vi "Loss-of-Comm Monitor.vi"(8 "Error In":errorcluster, 9 "Host to Ping":string, 11 "CTO!":refnum<notifier>) -> (0 "Error Out":errorcluster, 3 "CTO! Out":refnum<notifier>)   [LabVIEW 2018]
uses:
  Ping Reply Info.ctl
  Instance          10 28Saved   Loss-of-Comm Monitor .vi
  Instance           7 28Saved   Loss-of-Comm Monitor .vi
panel:
  in  "Tab":enum32{"Status", "Details"}(tab)
  out "CTO DownTime":dbl caption="Connection\nDown Time" format="%<%H:%M:%S>t"
  out "CTO Now?":bool caption="Connection:"
  out "PTO Current":bool caption="Current Status:\nLast Ping:"
  in  "Clear":bool
  out "CTO Time":timestamp caption="Connection Lost At:" format="%<%.1X\n%x>T"
  out "PTO Time":timestamp caption="Last Ping Lost At:" format="%<%.1X\n%x>T"
  out "CTO Latched?":bool caption="Connection \nTimed Out?"
  out "PTO Latched?":bool caption="Latched Status:\nPing Timed Out?"
  in  "Connection \nTimeout":u32=1000
  in  "Ping Timeout":i32=300
  in  "Restart":bool
  in  "Stop":bool
  out "Status":string
  out "Chart":i32(graph) caption="Ping Target: [10.6.6.1]"
  out "Last Error Out":errorcluster
  in  "ReTxDelay":u32=200
  out "RxCount":i32 caption="Packets Received"
  out "RxBytes":i32 caption="Bytes\nReceived\nBack"
  in  "Sequence Number":u16 format="%04x"
  out "Ping Reply Info":T1 {"Sequence" format="%04x"}
  out "Socket Out":u32 caption="Socket ID Obtained" format="%04x"
  out "Resolved Host IP":u32 format="%x"
  out "Bytes Sent":i32
  in  "Data Size in Bytes (32)":i32=8
  in  "TTL":u8=128 min=1
  out "LVT":u32
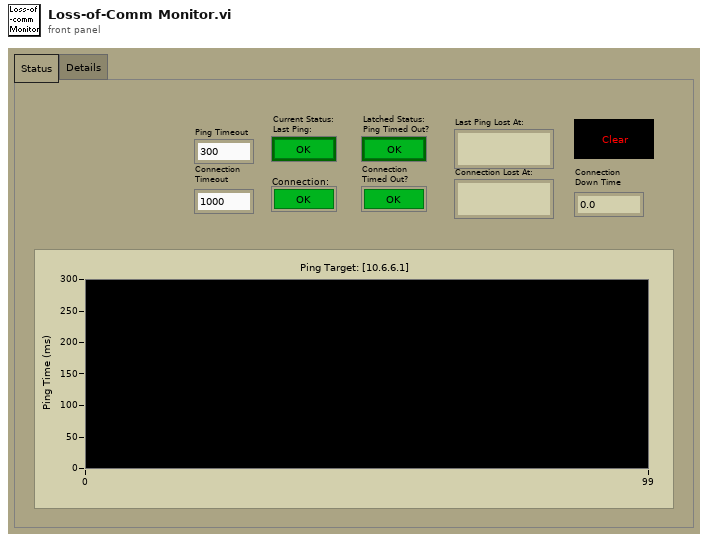
[diagram p1: front panel]
types:
  T1 = typedef "Ping Reply Info.ctl" = cluster{"Source Address":string, "Bytes":i32, "Sequence":u16, "Time (ms)":i32, "Hops":u8, "TTL Returned":u8, "Status":string}
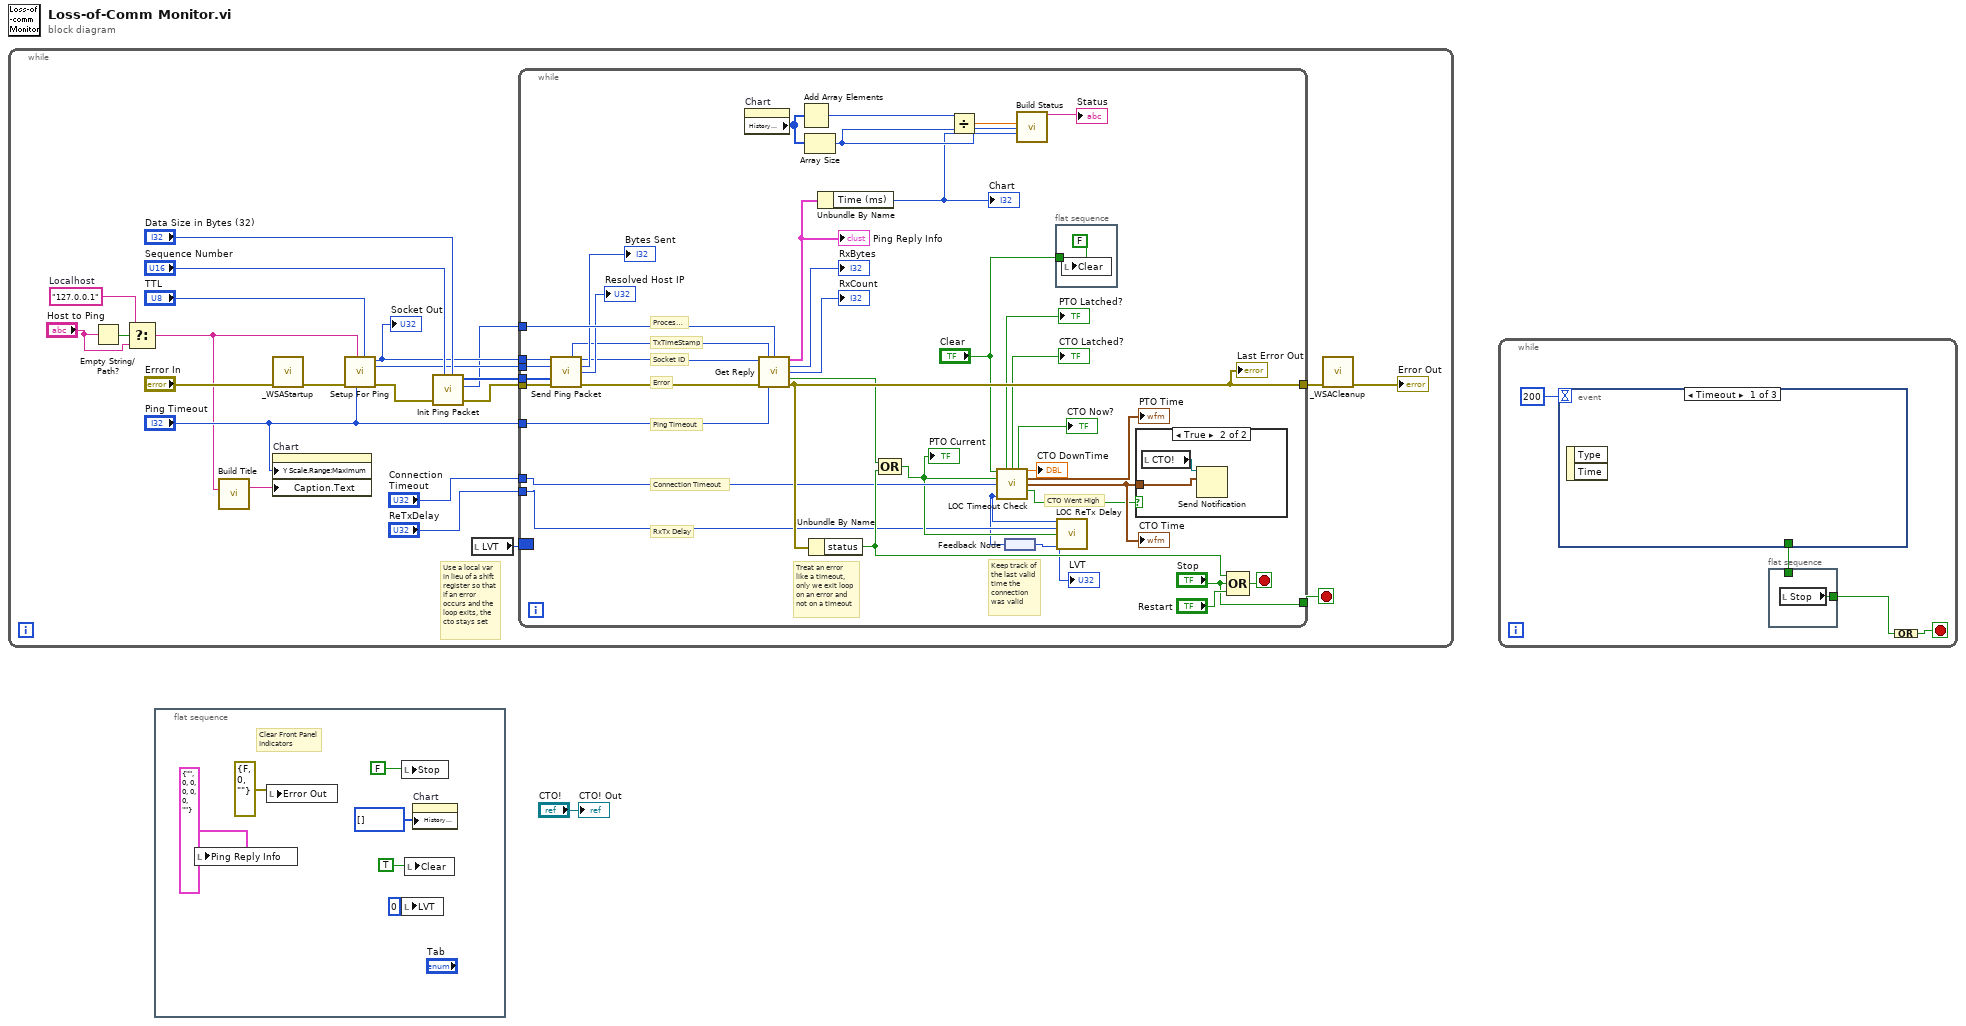
[diagram p0: block diagram]
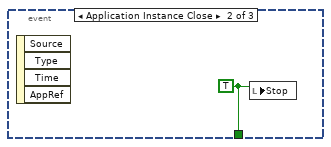
[diagram p2: hidden frame]
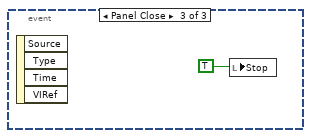
[diagram p3: hidden frame]
diagram:
  n1 = while {
    stop <- w11 stop-if-true
    w3 = "127.0.0.1"  # Localhost
    # "Use a local var\nin lieu of a shift\nregister so that\nif an error\noccurs and the\nloop exits, the\ncto stays set"
    n2 = Empty String/Path?(string/path="Host to Ping") -> (empty?=w5:bool)
    n3 = Select(t=w3, s=w5, f="Host to Ping") -> (s? t:f=w2:string)
    n4 = call "Build Title"("Host"=w2) -> ("Result"=w6:string)  [unwired: 13 in, 1 out]
    n5 = call "_WSAStartup.vi"("Error In"="Error In") -> ("Error out"=w24:errorcluster)  [unwired: 9 in, 1 out]
    n6 = property on="Chart" class="WFChart (strict)"("Y Scale.Range:Maximum"="Ping Timeout", "Caption.Text"=w6) -> ()  [unwired: 2 in, 2 out]
    n7 = call "Setup For Ping.vi"("TTL (U8)"="TTL", "Timeout (ms)"="Ping Timeout", "Host to Ping"=w2, "Error In"=w24) -> ("Error Out"=w23:errorcluster, "Resolved IP"=w16:u32, "Socket Out"=w15:u32)  [unwired: 5 in]
    "Socket Out" <- w15
    n8 = call "Init Ping Packet.vi"("Data Size in Bytes (32)"="Data Size in Bytes (32)", "Sequence Number"="Sequence Number", "Error In"=w23) -> ("Error Out"=w22:errorcluster, "ProcessID"=w13:u32, "Output Packet"=w14:u8[])  [unwired: 6 in]
    n9 = local read "LVT"() -> (w7:u32)
    n10 = while {
      tunnel: w22 -> [w63]
      tunnel: w16 -> [w62]
      tunnel: w15 -> [w61]
      tunnel: w14 -> [w60]
      tunnel: "Ping Timeout" -> [w59]
      tunnel: w13 -> [w58]
      tunnel: [w39] -> w12
      tunnel: ["Stop"] -> w11
      tunnel: "ReTxDelay" -> [w30]
      tunnel: "Connection \nTimeout" -> [w37]
      border: w7 -> [_]
      stop <- w49 stop-if-true
      # "CTO Went High"
      # "Keep track of\nthe last valid\ntime the\nconnection\nwas valid"
      # "RxTx Delay"
      # "Connection Timeout"
      # "Treat an error \nlike a timeout,\nonly we exit loop\non an error and\nnot on a timeout"
      # "Error"
      # "Ping Timeout"
      # "TxTimeStamp"
      # "Socket ID"
      # "ProcessID"
      n11 = call "Send Ping Packet.vi"("Socket To Use"=w61, "Resolved Host IP"=w62, "Packet to Send"=w60, "Error In"=w63) -> ("TxTimeStamp"=w51:u32, "Socket To Use Out"=w53:u32, "Bytes Sent"=→"Bytes Sent":i32, "Resolved Host IP Out"=→"Resolved Host IP":u32, "Error Out"=w52:errorcluster)  [unwired: 7 in]
      n12 = property on="Chart" class="WFChart (strict)"() -> ("History Data"=w47:i32[])  [unwired: 2 in, 2 out]
      n13 = call "Get Reply.vi"("Socket"=w53, "TxTimeStamp Alt"=w51, "ProcessID"=w58, "Error In"=w52, "Timeout (ms)"=w59) -> ("Ping Reply Info"=w50:T1, "RxBytes"=→"RxBytes":i32, "RxCount"=→"RxCount":i32, "Timed Out?"=w32:bool, "Error Out"=w39:errorcluster)  [unwired: 6 in]
      "Ping Reply Info" <- w50
      "Last Error Out" <- w39
      n14 = Add Array Elements(numeric array=w47) -> (sum=w48:i32)
      n15 = Array Size(array=w47) -> (size(s)=w44:i32)
      n16 = Unbundle By Name(w39) -> ("status"=w40:bool)
      n17 = Unbundle By Name(w50) -> ("Time (ms)"=w38:i32)
      "Chart" <- w38
      n18 = Compound Arithmetic op=OR(w32, w40) -> (w31:bool)
      "PTO Current" <- w31
      n19 = Divide(x=w48, y=w44) -> (x/y=w46:dbl)
      n20 = feedback #1() -> (w28:u32)
      n21 = call "LOC Timeout Check.vi"("Clear?"="Clear", "Ping Time Out?"=w31, "Connection Timeout"=w37, "Last Valid TimeStamp"=w28) -> ("PTO Latched"=→"PTO Latched?":bool, "CTO Latched"=→"CTO Latched?":bool, "CTO Current"=→"CTO Now?":bool, "CTO Total Time"=→"CTO DownTime":dbl, "Last PTO Time"=→"PTO Time":timestamp, "CTO Start Time"=w33:timestamp, "CTO Positive Edge"=w26:bool)  [unwired: 5 in]
      "CTO Time" <- w33
      n22 = call "Build Status"("Avg"=w46, "#"=w44, "Current"=w38) -> ("Result"=→"Status":string)  [unwired: 11 in, 1 out]
      n23 = flat-sequence {
        tunnel: "Clear" -> [_]
        frame #0 {
          n24 = local write "Clear"(FALSE ("Clear")) -> ()
        }
      }
      n25 = call "LOC ReTx Delay.vi"("Last Valid In"=w28, "ReTxDelay"=w30, "Ping Time Out?"=w31) -> ("Last Valid Out"=w27:u32)  [unwired: 12 in]
      "LVT" <- w27
      n26 = feedback-in #1(w27) -> ()
      n27 = case shown="True" w26 {
        tunnel: w33 -> [_ w65]
        frame False {
        }
        frame True {
          n28 = local read "CTO!"() -> (w64:refnum<notifier>)
          n29 = Send Notification(notification=w65, notifier=w64) -> ()  [unwired: 1 in, 2 out]
        }
      }
      n30 = Compound Arithmetic op=OR(w40, "Stop", "Restart") -> (w49:bool)
    }
    n31 = call "_WSACleanup.vi"("Error In"=w12) -> ("Error Out"=→"Error Out":errorcluster)  [unwired: 10 in]
  }
  n32 = flat-sequence {
    frame #0 {
      # "Clear Front Panel\nIndicators"
      n33 = local write "Ping Reply Info"(T1 {"Source Address"="", "Bytes"=0, "Sequence"=0, "Time (ms)"=0, "Hops"=0, "TTL Returned"=0, "Status"=""} ("Ping Reply Info")) -> ()
      n34 = local write "Error Out"(errorcluster {"status"=FALSE, "code"=0, "source"=""} ("Error Out")) -> ()
      n35 = local write "Stop"(FALSE ("End")) -> ()
      n36 = local write "LVT"(u32 0 ("LVT")) -> ()
      n37 = local write "Clear"(TRUE ("Clear")) -> ()
      n38 = property on="Chart" class="WFChart (strict)"("History Data"=i32[] []) -> ()  [unwired: 2 in, 2 out]
    }
  }
  n39 = while {
    stop <- w76 stop-if-true
    n40 = event shown="[0] Timeout" {
      selector: _ -> [_ _ _]
      dyn-events: _ -> [_ _ _]
      timeout: 200 -> [_ _ _]
      tunnel: [_ w78 _] -> w73
      event Timeout {
        n41 = event-data() -> ()  [unwired: 1 in, 2 out]
      }
      event Application Instance Close {
        w78 = TRUE ("End")
        n42 = event-data() -> ()  [unwired: 1 in, 4 out]
        n43 = local write "Stop"(w78) -> ()
      }
      event Panel Close {
        n44 = event-data() -> ()  [unwired: 1 in, 4 out]
        n45 = local write "Stop"(TRUE ("End")) -> ()
      }
    }
    n46 = flat-sequence {
      tunnel: [w77] -> w74
      tunnel: w73 -> [_]
      frame #0 {
        n47 = local read "Stop"() -> (w77:bool)
      }
    }
    n48 = Compound Arithmetic op=OR(w74) -> (w76:bool)
  }
  "CTO! Out" <- "CTO!"
